vi "move Y.vi"(9 "x mm":dbl, 10 "Vitesse":dbl, 11 "y mm":dbl) -> (2 "Y Speed":i32, 3 "Numeric 2":i32)   [LabVIEW 2016]
uses:
  Variable globale.vi
  <userlib>/ICNC/ICNC2.lvlib
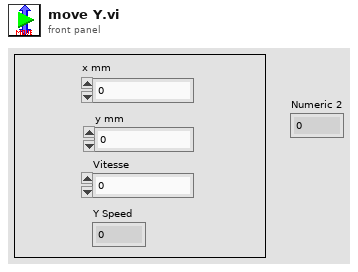
[diagram p1: front panel]
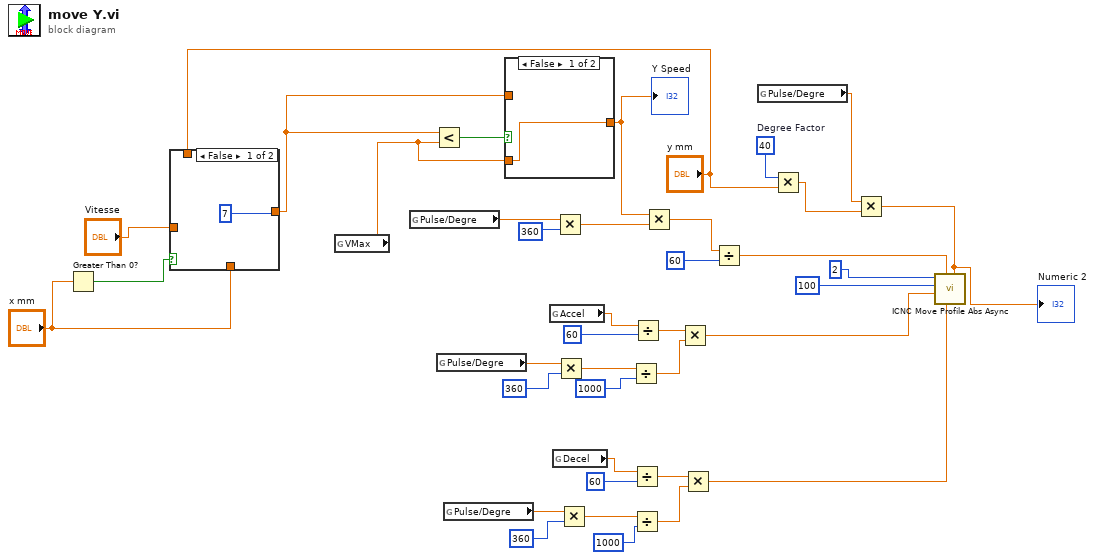
[diagram p0: block diagram]
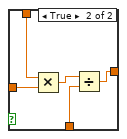
[diagram p2: hidden frame]
diagram:
  w10 = 40  # Degree Factor
  n1 = Greater Than 0?(x="x mm") -> (x > 0?=w3:bool)
  n2 = case shown="False" w3 {
    tunnel: "x mm" -> [_ w41]
    tunnel: [7 w40] -> w2
    tunnel: "y mm" -> [_ w43]
    tunnel: "Vitesse" -> [_ w44]
    frame False {
    }
    frame True {
      n3 = Multiply(x=w43, y=w44) -> (x*y=w42:dbl)
      n4 = Divide(x=w42, y=w41) -> (x/y=w40:dbl)
    }
  }
  n5 = global read "Variable globale.vi" "VMax"() -> (w19:dbl)
  n6 = global read "Variable globale.vi" "Pulse/Degre"() -> (w27:dbl)
  n7 = Less?(x=w2, y=w19) -> (x < y?=w20:bool)
  n8 = global read "Variable globale.vi" "Pulse/Degre"() -> (w36:dbl)
  n9 = global read "Variable globale.vi" "Pulse/Degre"() -> (w30:dbl)
  n10 = case shown="False" w20 {
    tunnel: w2 -> [_ w46]
    tunnel: w19 -> [w45 _]
    tunnel: [w45 w46] -> w1
    frame False {
    }
    frame True {
    }
  }
  "Y Speed" <- w1
  n11 = global read "Variable globale.vi" "Accel"() -> (w25:dbl)
  n12 = global read "Variable globale.vi" "Decel"() -> (w15:dbl)
  n13 = Multiply(x=w27, y=360) -> (x*y=w16:dbl)
  n14 = Multiply(x=w36, y=360) -> (x*y=w18:dbl)
  n15 = Multiply(x=w30, y=360) -> (x*y=w17:dbl)
  n16 = Divide(x=w18, y=1000) -> (x/y=w37:dbl)
  n17 = Divide(x=w15, y=60) -> (x/y=w32:dbl)
  n18 = Divide(x=w17, y=1000) -> (x/y=w31:dbl)
  n19 = Divide(x=w25, y=60) -> (x/y=w23:dbl)
  n20 = Multiply(x=w1, y=w16) -> (x*y=w22:dbl)
  n21 = Multiply(x=w23, y=w37) -> (x*y=w12:dbl)
  n22 = Multiply(x=w32, y=w31) -> (x*y=w11:dbl)
  n23 = Divide(x=w22, y=60) -> (x/y=w8:dbl)
  n24 = global read "Variable globale.vi" "Pulse/Degre"() -> (w21:dbl)
  n25 = Multiply(x=w10, y="y mm") -> (x*y=w9:dbl)
  n26 = Multiply(x=w21, y=w9) -> (x*y=w7:dbl)
  "Numeric 2" <- w7
  n27 = call "ICNC Move Profile Abs Async.vi"("Position"=w7, "Decel"=w11, "Speed"=w8, "Accel"=w12, "FStartStop"=100, "Axe"=2) -> ()  [unwired: 4 in, 2 out]
